vi "ReplaceSubVINode.vi"(5 "Old File Name":string, 7 "New File Name":string, 8 "error in (no error)":errorcluster, 11 "VI Refnum In":refnum<vi>) -> (0 "error out":errorcluster, 3 "VI Refnum Out":refnum<vi>, 4 "Replaced":bool)   [LabVIEW 2024]
uses:
  <vilib>/Utility/traverseref.llb/TRef TravTarget.ctl
  <vilib>/Utility/traverseref.llb/VI Scripting - Traverse.lvlib
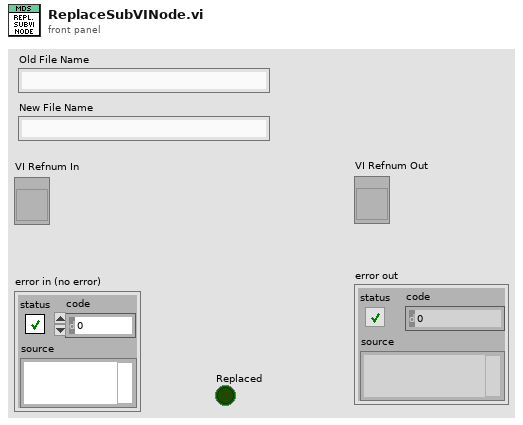
[diagram p1: front panel]
types:
  T1 = typedef "TRef TravTarget.ctl" = enum16{"FP", "BD", "Other"}
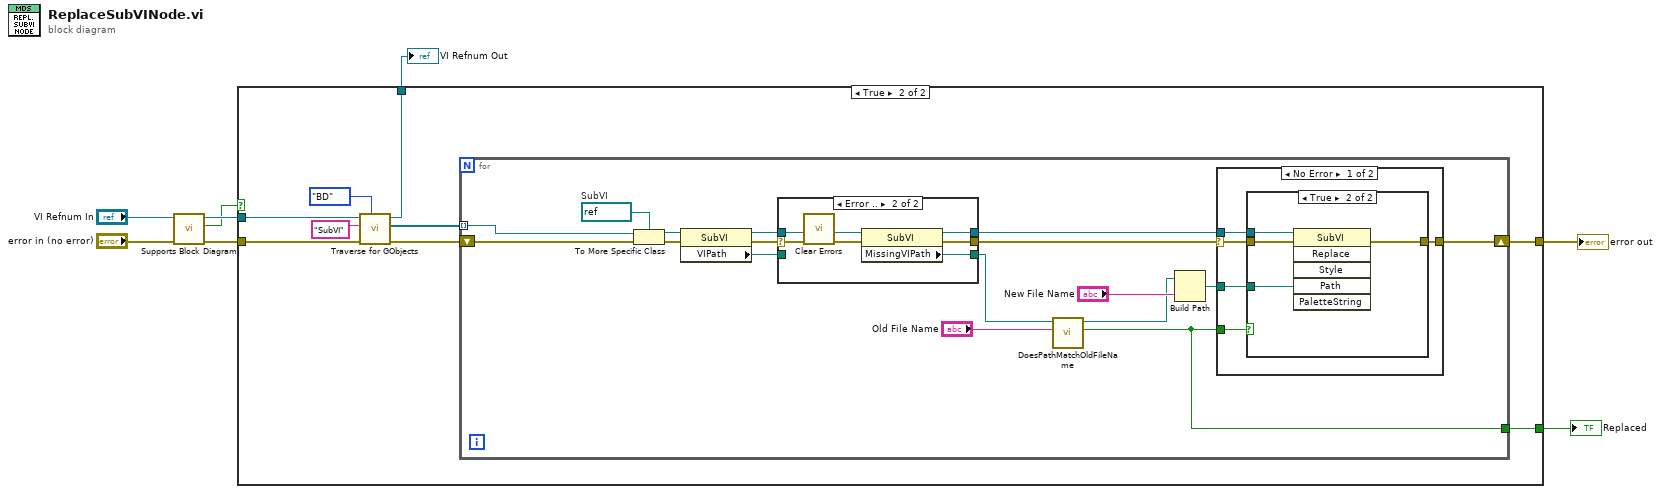
[diagram p0: block diagram]
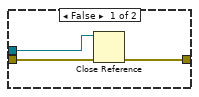
[diagram p3: hidden frame]
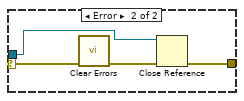
[diagram p4: hidden frame]
diagram:
  n1 = call "Supports Block Diagram.vi"("error in (no error)"="error in (no error)", "vi in"="VI Refnum In") -> ("error out"=w3:errorcluster, "has block diagram"=w1:bool, "vi out"=w2:refnum<vi>)  [unwired: 7 in]
  n2 = case shown="True" w1 {
    tunnel: w2 -> [w9 w15]
    tunnel: w3 -> [w10 w14]
    tunnel: [_ w13] -> w8
    tunnel: [w10 w12] -> w7
    tunnel: [w9 w11] -> w6
    frame False {
    }
    frame True {
      n3 = call <vilib>:"Traverse for GObjects.vi"("Traverse Target"=TRef_TravTarget."BD", "error in (no error)"=w14, "Class Name"="SubVI", "VI Refnum"=w15) -> ("error out"=w18:errorcluster, "References"=w19:refnum<vi>[], "dup VI Refnum"=w11:refnum<vi>)  [unwired: 4 in, 1 out]
      n4 = for {
        shift-right: [w28] -> w12
        shift-left: w18 -> [w32]
        tunnel: w19 -> [w33] mode=indexing
        tunnel: [w21] -> w13
        w34 = refnum<vi> refnum  # SubVI
        n5 = To More Specific Class(target class=w34, reference=w33, error in=w32) -> (specific class reference=w35:refnum<vi>, error out=w36:errorcluster)
        n6 = property class="SubVI"(reference=w35, error in=w36) -> (reference out=w30:refnum<vi>, error out=w29:errorcluster, "VIPath"=w31:path)
        n7 = case shown="Error .." w29 {
          selector: w29 -> [w55 w61]
          tunnel: w31 -> [w54 _]
          tunnel: [w55 w59] -> w26
          tunnel: w30 -> [w53 w58]
          tunnel: [w53 w57] -> w27
          tunnel: [w54 w56] -> w23
          frame No Error {
          }
          frame Error {
            n8 = call <vilib>:"Clear Errors.vi"("error in (no error)"=w61) -> ("error out"=w60:errorcluster)  [unwired: 5 in, 1 out]
            n9 = property class="SubVI"(reference=w58, error in=w60) -> (reference out=w57:refnum<vi>, error out=w59:errorcluster, "MissingVIPath"=w56:path)
          }
        }
        n10 = call "DoesPathMatchOldFileName.vi"("Old File Name"="Old File Name", "File Path"=w23) -> ("Match Found"=w21:bool, "Parent Directory"=w20:path)  [unwired: 8 in]
        n11 = Build Path(base path=w20, name or relative path="New File Name") -> (appended path=w25:path)
        n12 = case shown="No Error" w26 {
          selector: w26 -> [w37 w52]
          tunnel: w25 -> [w41 _]
          tunnel: w21 -> [w40 _]
          tunnel: [w39 w50] -> w28
          tunnel: w27 -> [w38 w49]
          frame No Error {
            n13 = case shown="True" w40 {
              tunnel: w41 -> [_ w48]
              tunnel: w37 -> [w44 w47]
              tunnel: [w43 w45] -> w39
              tunnel: w38 -> [w42 w46]
              frame False {
                n14 = Close Reference(reference=w42, error in (no error)=w44) -> (error out=w43:errorcluster)
              }
              frame True {
                n15 = invoke class="SubVI" method="Replace"(reference=w46, error in=w47, "Path"=w48) -> (error out=w45:errorcluster)  [unwired: 3 in, 5 out]
              }
            }
          }
          frame Error {
            n16 = call <vilib>:"Clear Errors.vi"("error in (no error)"=w52) -> ("error out"=w51:errorcluster)  [unwired: 5 in, 1 out]
            n17 = Close Reference(reference=w49, error in (no error)=w51) -> (error out=w50:errorcluster)
          }
        }
      }
    }
  }
  "error out" <- w7
  "Replaced" <- w8
  "VI Refnum Out" <- w6
